vi "calculator.vi"() -> ()   [LabVIEW 2013]
uses:
  <vilib>/Utility/file.llb/Read From Spreadsheet File (DBL).vi
  <vilib>/express/express arith-compare/Formula/XNode/ExpressFormulaBlockNode.xnode
panel:
  out "XY Graph":cluster{"Y":dbl[], "Y":dbl[]}[](graph)
  out "Laser Bandwidth (nm)":dbl
  out "Converged?":bool
  out "Iterations":i32
  out "Initial Length cm":dbl
  in  "?":bool
  in  "?":bool
  out "Limiting Length cm":dbl
  in  "Laser Width (fs)":dbl
  in  "Dispersion (mm)":sgl
  in  "Prism Material":sgl(ring) items=["FS", "Lak21", "SF10", "BK7"]
  in  "Wavelength":sgl(ring) items=["400", "450", "500", "550", "600", "650", "700", "750", "800", "850", ""]
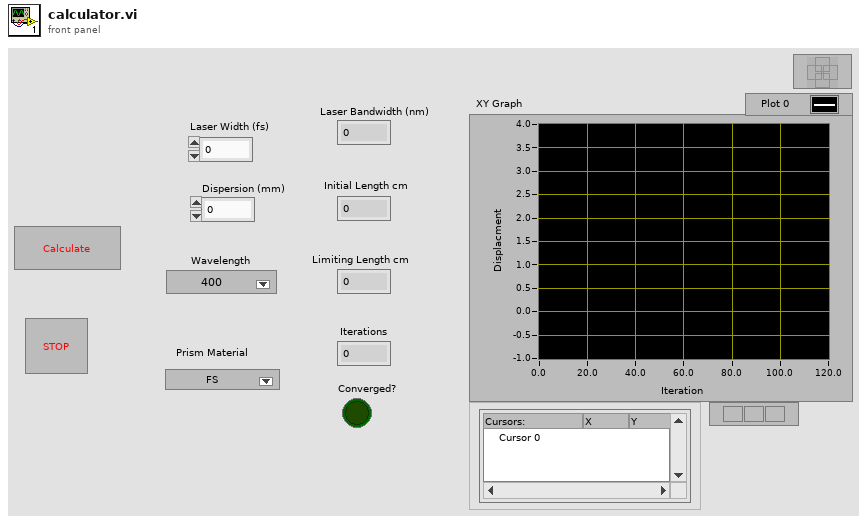
[diagram p1: front panel]
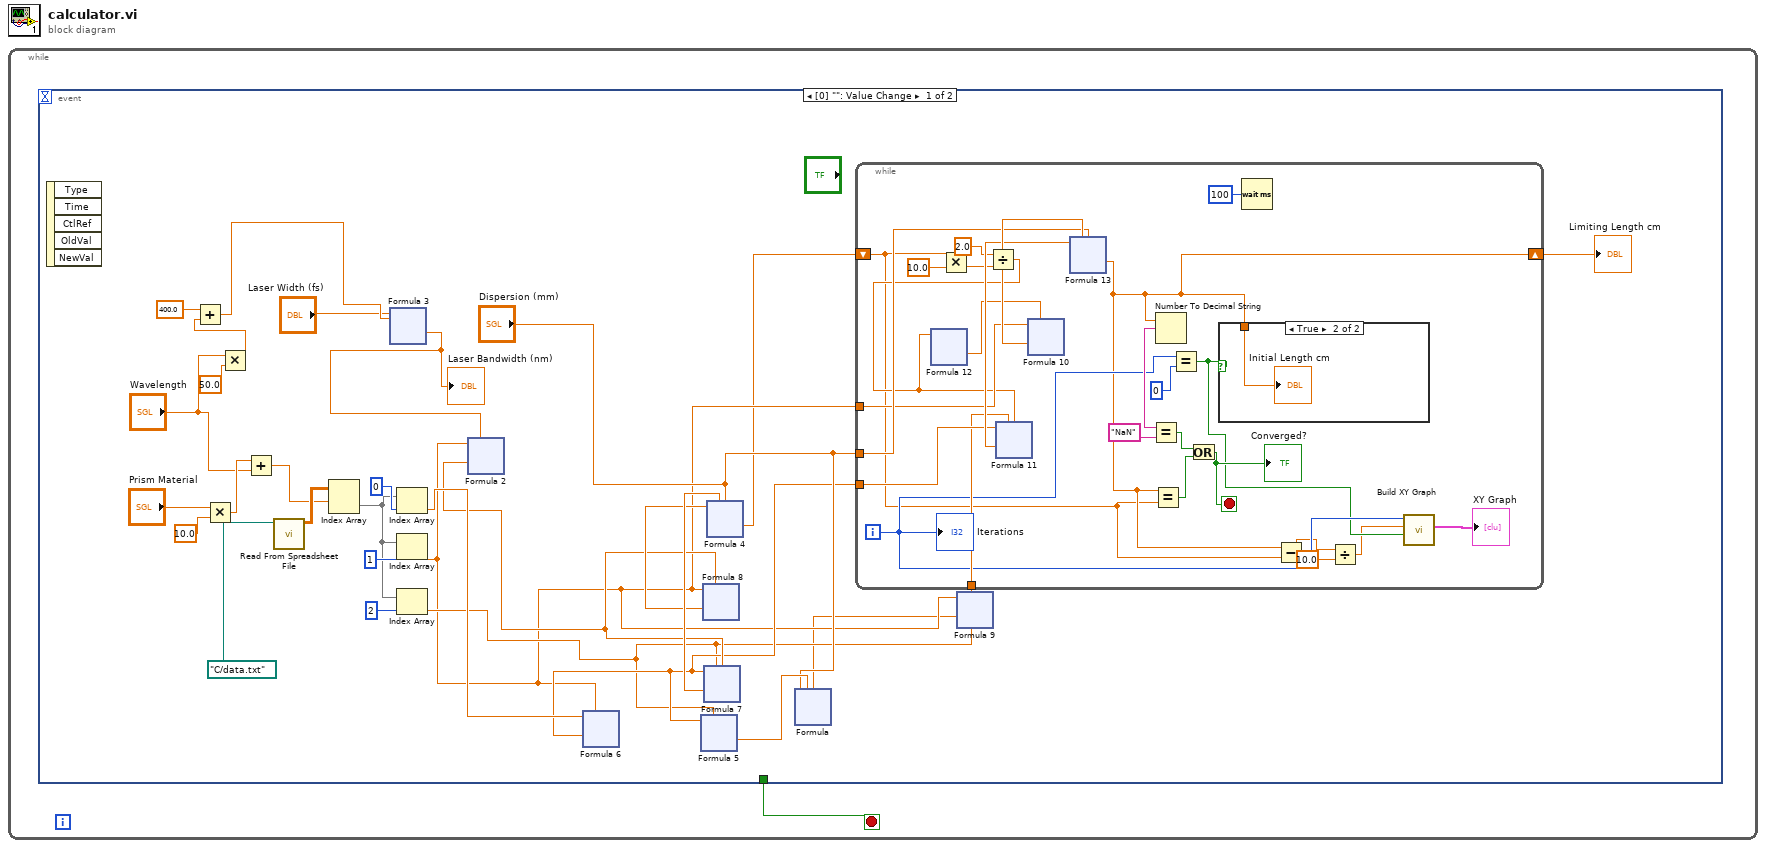
[diagram p0: block diagram]
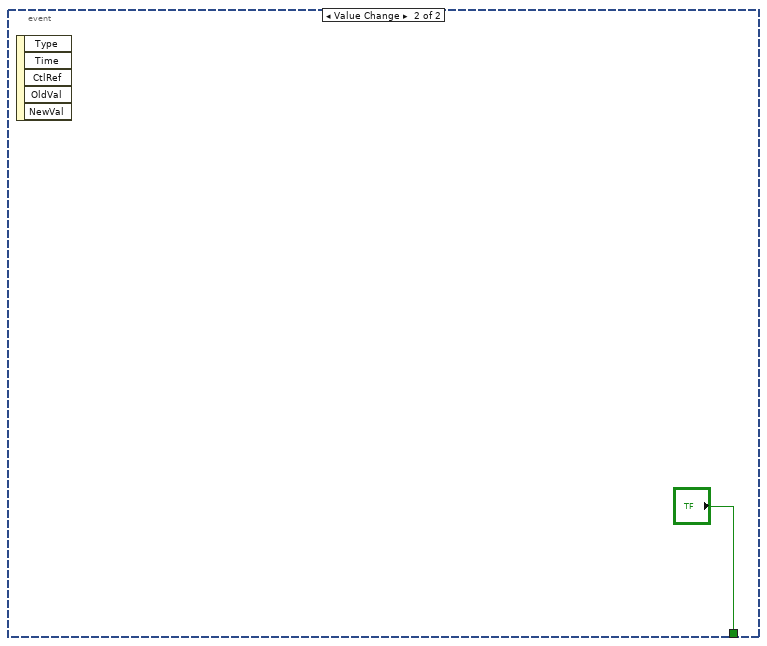
[diagram p3: hidden frame]
diagram:
  n1 = while {
    stop <- w1 stop-if-true
    n2 = event shown="[0] \"\": Value Change" {
      selector: _ -> [_ _]
      dyn-events: _ -> [_ _]
      timeout: _ -> [_ _]
      tunnel: [_ "?"] -> w1
      event Value Change {
        n3 = event-data() -> ()  [unwired: 1 in, 5 out]
        n4 = Multiply(x="Prism Material", y=sgl 10.0) -> (x*y=w28:sgl)
        n5 = Multiply(x="Wavelength", y=sgl 50.0) -> (x*y=w6:sgl)
        n6 = Add(x=400.0, y=w6) -> (x+y=w5:dbl)
        n7 = Add(x=w28, y="Wavelength") -> (x+y=w26:sgl)
        n8 = call-poly <vilib>:"Read From Spreadsheet File.vi"("file path (dialog if empty)"=path "C:/data.txt") -> ("all rows"=w27:dbl[][])  [unwired: 6 in, 4 out]
        n9 = Index Array(array=w27, index (row)=w26) -> (element=w23:dbl[])  [unwired: 1 in]
        n10 = xnode "Formula 3"("X1"="Laser Width (fs)", "X2"=w5) -> ("Result"=w19:dbl)  [unwired: 1 in, 1 out]
        "Laser Bandwidth (nm)" <- w19
        n11 = Index Array(array=w23, index=0) -> (element=w20:dbl)
        n12 = Index Array(array=w23, index=1) -> (element=w11:dbl)
        n13 = Index Array(array=w23, index=2) -> (element=w12:dbl)
        n14 = xnode "Formula 2"("X1"=w11, "X2"=w19) -> ("Result"=w15:dbl)  [unwired: 1 in, 1 out]
        n15 = xnode "Formula 6"("X1"=w20, "X2"=w11) -> ("Result"=w13:dbl)  [unwired: 1 in, 1 out]
        n16 = xnode "Formula 5"("X1"=w13, "X2"=w12) -> ("Result"=w17:dbl)  [unwired: 1 in, 1 out]
        n17 = xnode "Formula 8"("X1"=w11, "X2"=w15) -> ("Result"=w16:dbl)  [unwired: 1 in, 1 out]
        n18 = xnode "Formula 7"("X1"=w13, "X2"=w12, "X3"=w15) -> ("Result"=w18:dbl)  [unwired: 1 in, 1 out]
        n19 = xnode "Formula 4"("X1"=w16, "X2"=w18, "X3"="Dispersion (mm)") -> ("Result"=w10:dbl)  [unwired: 1 in, 1 out]
        n20 = while {
          tunnel: "Dispersion (mm)" -> [w54]
          tunnel: w13 -> [w53]
          tunnel: w12 -> [w52]
          tunnel: w11 -> [w51]
          shift-right: [w37] -> w3
          shift-left: w10 -> [w34]
          i -> [w38]
          stop <- w36 stop-if-true
          n21 = Multiply(x=w34, y=10.0) -> (x*y=w48:dbl)
          n22 = Divide(x=2.0, y=w48) -> (x/y=w46:dbl)
          n23 = xnode "Formula 12"("X1"=w46) -> ("Result"=w47:dbl)  [unwired: 1 in, 1 out]
          n24 = xnode "Formula 11"("X1"=w53, "X2"=w52, "X3"=w46) -> ("Result"=w55:dbl)  [unwired: 1 in, 1 out]
          n25 = xnode "Formula 10"("X1"=w51, "X2"=w47) -> ("Result"=w56:dbl)  [unwired: 1 in, 1 out]
          n26 = xnode "Formula 13"("X1"=w55, "X2"=w56, "X3"=w54) -> ("Result"=w37:dbl)  [unwired: 1 in, 1 out]
          n27 = Equal?(x=w37, y=w34) -> (x = y?=w42:bool)
          n28 = Number To Decimal String(number=w37) -> (decimal integer string=w43:string)  [unwired: 1 in]
          n29 = Equal?(x=w43, y="NaN") -> (x = y?=w41:bool)
          n30 = Equal?(x=w38, y=0) -> (x = y?=w35:bool)
          n31 = Or(x=w41, y=w42) -> (x .or. y?=w36:bool)
          "Converged?" <- w36
          n32 = case shown="True" w35 {
            tunnel: w37 -> [_ w57]
            frame False {
            }
            frame True {
              "Initial Length cm" <- w57
            }
          }
          n33 = Wait (ms)(milliseconds to wait=u32 100) -> ()  [unwired: 1 out]
          n34 = Subtract(x=w37, y=w34) -> (x-y=w32:dbl)
          n35 = Divide(x=w32, y=10.0) -> (x/y=w31:dbl)
          n36 = call "Build XY Graph"("Reset"=w35, "Y Input"=w31, "X Input"=w38) -> ("XY Graph"=→"XY Graph":cluster{"X":dbl[], "Y":dbl[]}[])  [unwired: 7 in, 1 out]
          "Iterations" <- w38
        }
        "Limiting Length cm" <- w3
        n37 = xnode "Formula 9"("X1"=w11) -> ("Result"=w2:dbl)  [unwired: 1 in, 1 out]
        n38 = xnode "Formula"("X1"="Dispersion (mm)", "X2"=w17, "X3"=w2) -> ()  [unwired: 1 in, 2 out]
      }
      event Value Change {
        n39 = event-data() -> ()  [unwired: 1 in, 5 out]
      }
    }
  }
